vi "spurverfolgung_mit_punkten.vi"() -> ()   [LabVIEW 2014]
uses:
  <vilib>/userdefined/High Color/IMAQdx.ctl
  <vilib>/vision/driver/NI_Vision_Acquisition_Software.lvlib
  <vilib>/vision/NI_Vision_Development_Module.lvlib
panel:
  out "x":dbl
  out "y":dbl
  out "output array":dbl[][](array[numeric])
  in  "millisecond multiple":u32
  in  "größe":sgl
  out "date/time string":string
  in  "file path (dialog if empty)":path
  out "Y Resolution":i32
  out "X Resolution":i32
  in  "Template File Path (Pattern Matching 1)":path=path "C:/Users/stdekrol/Videos/patter_neu.png"
  out "Position":cluster{"x":sgl, "y":sgl}
  out "ROI":T1
  in  "Advanced Options (Pattern Matching 1)":cluster{"Item":u16, "Value":dbl}[](array[cluster])=[{"Item"=0, "Value"=10.0}, {"Item"=2, "Value"=2.0}, {"Item"=5, "Value"=300.0}, {"Item"=6, "Value"=3.0}, {"Item"=7, "Value"=5.0}, {"Item"=8, "Value"=2.0}, {"Item"=1, "Value"=1.0}, {"Item"=3, "Value"=20.0}, {"Item"=4, "Value"=0.0}] {"Item" items=["LD Sampling - Minimum Constrast"=0, "LD Sampling - Enable Subpixel Accuracy"=1, "LD Sampling - Search Strategy"=2, "LD Sampling - Subpixel Iterations"=3, "LD Sampling - Subpixel Tolerance"=4, "LD Sampling - Initial Match List Length"=5, "LD Sampling - Match List Reduction Factor"=6, "LD Sampling - Initial Step Size"=7, "LD Sampling - Intermediate Angular Accuracy"=8, "-"=9, "Pyramid - Max Pyramid Level"=100, "Pyramid - Minimum Contrast"=102, "Pyramid - Enable Subpixel Accuracy"=103, "Pyramid - Subpixel Iterations"=104, "Pyramid - Subpixel Tolerance"=105, "Pyramid - Initial Match List Length"=106, "Pyramid - Match List Reduction Factor"=107, "Pyramid - Intermediate Angular Accuracy"=108, "Pyramid - Process Border Matches"=109, "Pyramid - Min Match Separation Distance"=111, "Pyramid - Min Match Separation Angle"=112, "Pyramid - Max Match Overlap"=113, "Pyramid - Max Cache in MB"=114, "Pyramid - Clear Cache"=115]}
  in  "Parameters (Pattern Matching 1)":T2={"Number of Matches Requested"=1, "Minimum Match Score"=500.0, "Angle Ranges"=[{"Start Angle"=-180.0, "End Angle"=180.0}, {"Start Angle"=0.0, "End Angle"=360.0}]}
  in  "Algorithm (Pattern Matching 1)":i32(ring)=1 items=["All", "Low Discrepancy Sampling", "Grayscale Value Pyramid", "Gradients Pyramid"]
  out "Frame rate":dbl
  out "Matches (Pattern Matching 1)":T3(array[cluster]) {"Bounding Box"."y" format="%.2f"; "Bounding Box"."x" format="%.2f"; "Position"."y" format="%.2f"; "Position"."x" format="%.2f"; "Score" format="%.2f"; "Scale" format="%.2f"; "Angle" format="%.2f"}
  out "Number of Matches (Pattern Matching 1)":i32
  in  "stop":bool
  in  "Replace Value (1)":sgl=255.0 format="%.2f"
  in  "Threshold Limits":cluster{"Lower value":sgl, "Upper value":sgl}={"Lower value"=0.0, "Upper value"=150.0} {"Upper value" format="%.2f"; "Lower value" format="%.2f"}
  in  "Method (clustering)":i32(ring) items=["clustering", "entropy", "metric", "moments", "inter-class variance"]
  in  "Look For (Bright Objects)":u32(ring) items=["Bright Objects", "Dark Objects"]
  out "Threshold Image 2":T4(plugin-control)
  in  "Keep/Replace Value (Replace)":bool=TRUE
  out "Image 2":T4(plugin-control)
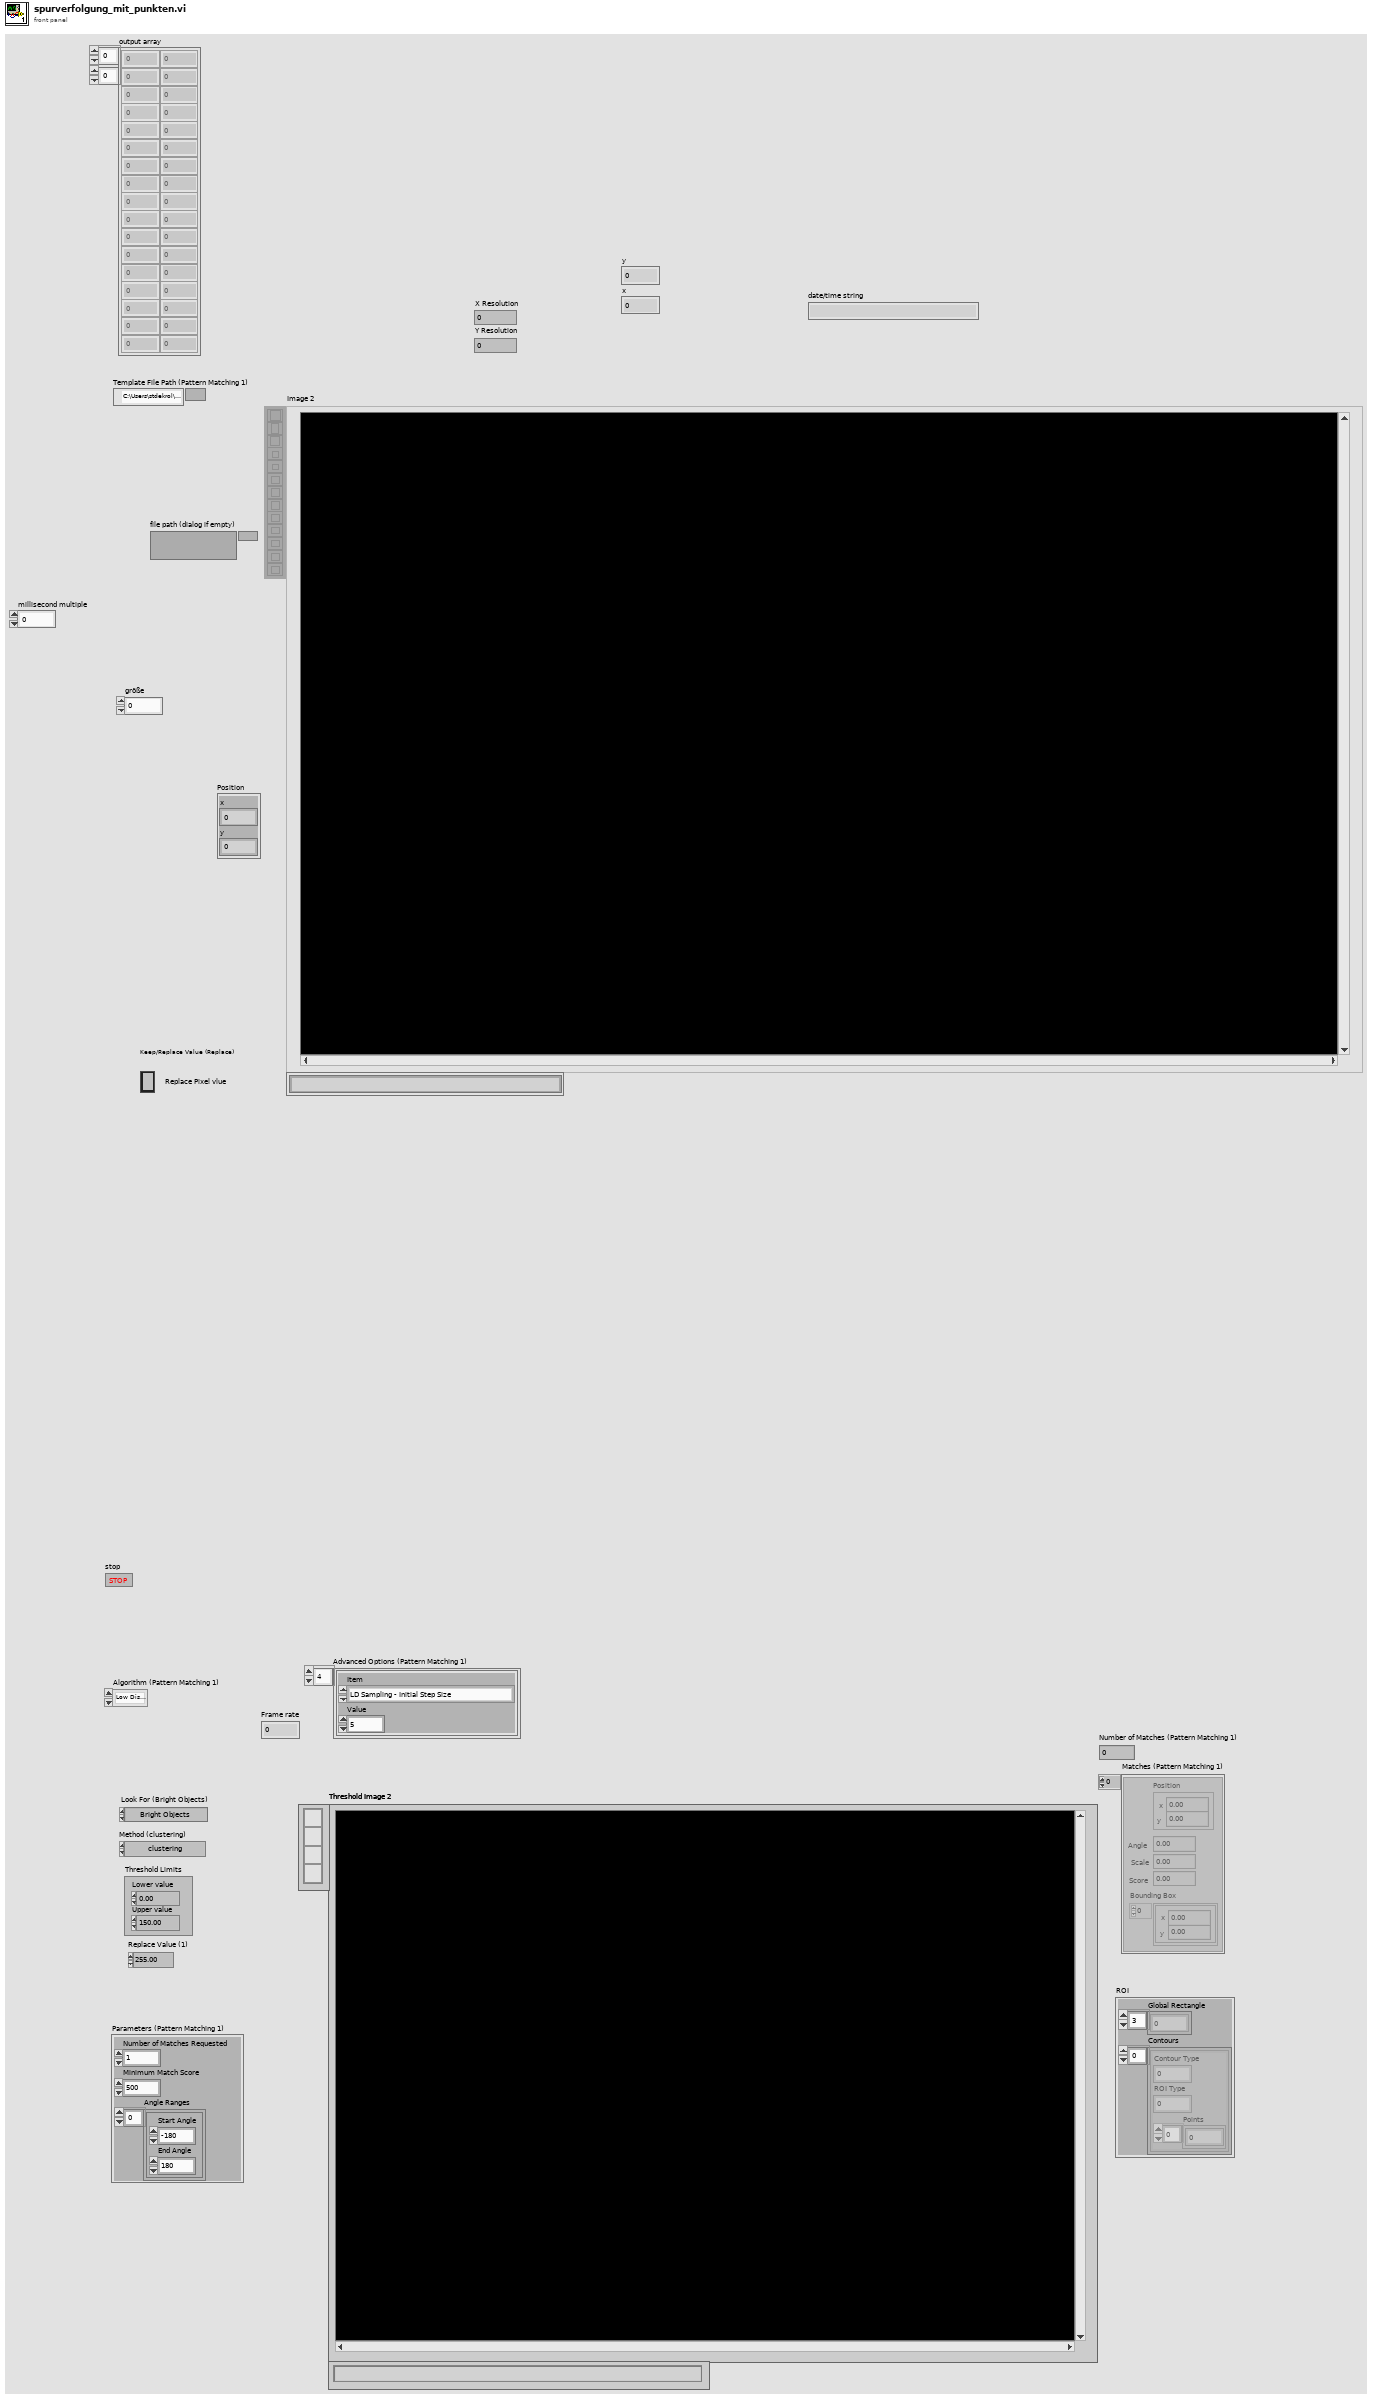
[diagram p1: front panel]
types:
  T1 = cluster{"Global Rectangle":i32[], "Contours":cluster{"Contour Type":u32, "ROI Type":u32, "Points":i32[]}[]}
  T2 = cluster{"Number of Matches Requested":i32, "Minimum Match Score":sgl, "Angle Ranges":cluster{"Start Angle":sgl, "End Angle":sgl}[]}
  T3 = cluster{"Position":cluster{"x":sgl, "y":sgl}, "Angle":sgl, "Scale":sgl, "Score":sgl, "Bounding Box":cluster{"x":sgl, "y":sgl}[]}[]
  T4 = typedef "IMAQ Image.ctl" = refnum<image>
  T5 = enum16{"open", "replace", "create", "open or create", "replace or create", "replace or create with confirmation"}
  T6 = typedef "Image Type" = u32
  T7 = typedef "IMAQdx.ctl" = refnum<k21>
  T8 = cluster{"Matches (Pattern Matching 1)[0]":cluster{"Position":cluster{"x":sgl, "y":sgl}, "Angle":sgl, "Scale":sgl, "Score":sgl, "Bounding Box":cluster{"x":sgl, "y":sgl}[]}, "Matches (Pattern Matching 1)[1]":cluster{"Position":cluster{"x":sgl, "y":sgl}, "Angle":sgl, "Scale":sgl, "Score":sgl, "Bounding Box":cluster{"x":sgl, "y":sgl}[]}, "Matches (Pattern Matching 1)[2]":cluster{"Position":cluster{"x":sgl, "y":sgl}, "Angle":sgl, "Scale":sgl, "Score":sgl, "Bounding Box":cluster{"x":sgl, "y":sgl}[]}, "Matches (Pattern Matching 1)[3]":cluster{"Position":cluster{"x":sgl, "y":sgl}, "Angle":sgl, "Scale":sgl, "Score":sgl, "Bounding Box":cluster{"x":sgl, "y":sgl}[]}, "Matches (Pattern Matching 1)[4]":cluster{"Position":cluster{"x":sgl, "y":sgl}, "Angle":sgl, "Scale":sgl, "Score":sgl, "Bounding Box":cluster{"x":sgl, "y":sgl}[]}, "Matches (Pattern Matching 1)[5]":cluster{"Position":cluster{"x":sgl, "y":sgl}, "Angle":sgl, "Scale":sgl, "Score":sgl, "Bounding Box":cluster{"x":sgl, "y":sgl}[]}, "Matches (Pattern Matching 1)[6]":cluster{"Position":cluster{"x":sgl, "y":sgl}, "Angle":sgl, "Scale":sgl, "Score":sgl, "Bounding Box":cluster{"x":sgl, "y":sgl}[]}, "Matches (Pattern Matching 1)[7]":cluster{"Position":cluster{"x":sgl, "y":sgl}, "Angle":sgl, "Scale":sgl, "Score":sgl, "Bounding Box":cluster{"x":sgl, "y":sgl}[]}, "Matches (Pattern Matching 1)[8]":cluster{"Position":cluster{"x":sgl, "y":sgl}, "Angle":sgl, "Scale":sgl, "Score":sgl, "Bounding Box":cluster{"x":sgl, "y":sgl}[]}}
  T9 = cluster{"Position":cluster{"x":sgl, "y":sgl}, "Angle":sgl, "Scale":sgl, "Score":sgl, "Bounding Box":cluster{"x":sgl, "y":sgl}[]}
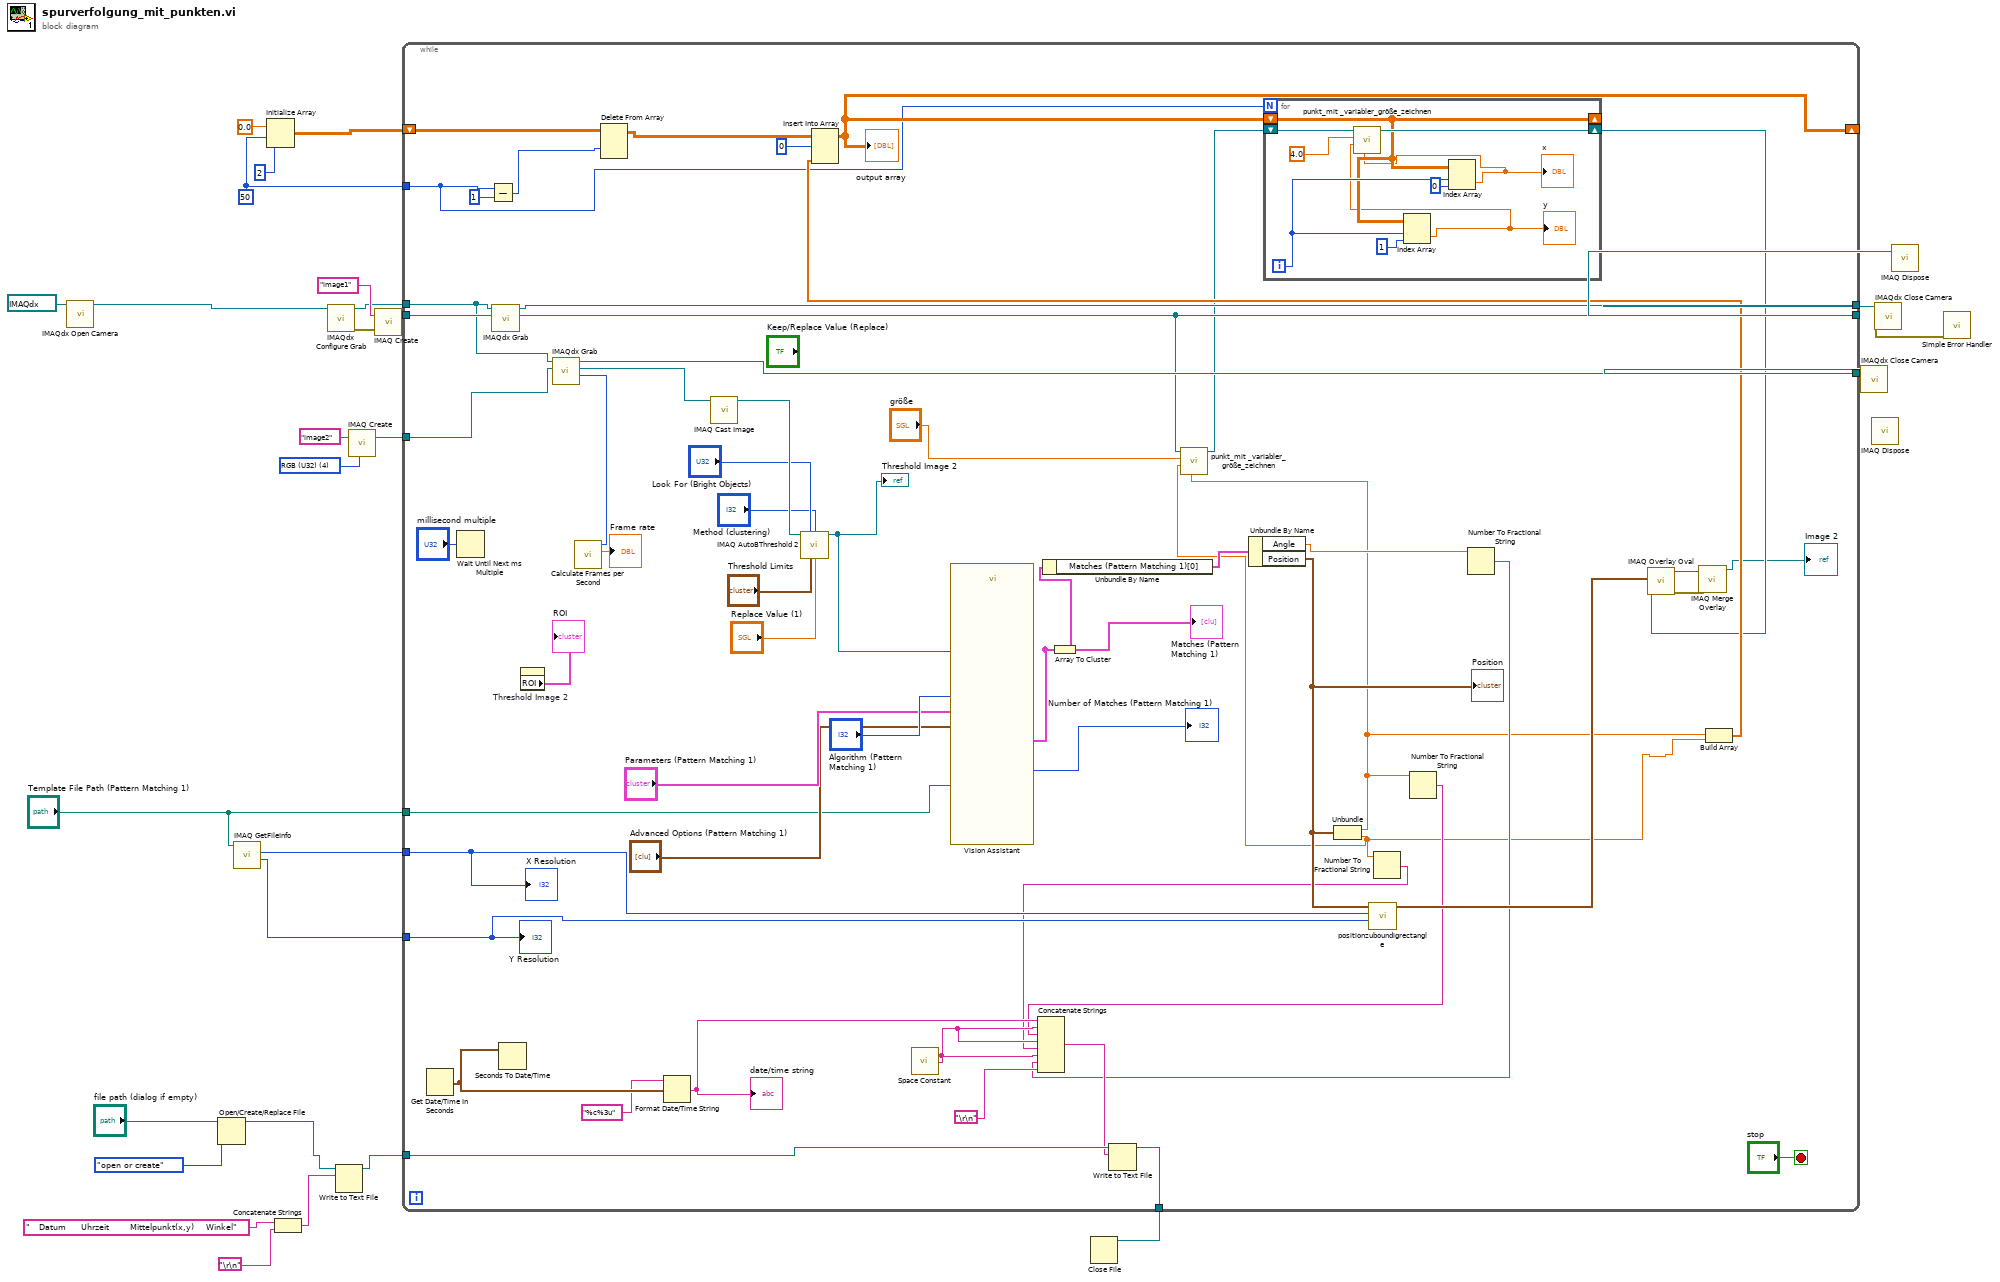
[diagram p0: block diagram]
diagram:
  w1 = 50 ("dimension size")
  w16 = T6 4 items=["Grayscale (U8)", "Grayscale (I16)", "Grayscale (SGL)", "Complex (CSG)", "RGB (U32)", "HSL (U32)", "RGB (U64)", "Grayscale (U16)"] ("Image Type")
  n1 = call <vilib>:"IMAQdx Open Camera.vi"("Session In"=T7 "cam0") -> ("Session Out"=w21:T7)  [unwired: 9 in, 1 out]
  n2 = Open/Create/Replace File(file path (use dialog)="file path (dialog if empty)", operation (0:open)=T5."open or create") -> (refnum out=w9:refnum<file>)  [unwired: 4 in, 2 out]
  n3 = call "IMAQ GetFileInfo"("File Path"="Template File Path (Pattern Matching 1)") -> ("Y Resolution"=w13:i32, "X Resolution"=w14:i32)  [unwired: 4 in, 5 out]
  n4 = Initialize Array "Initialize Array"(0.0 ("element"), w1, 2 ("dimension size")) -> (w3:dbl[][])
  n5 = Concatenate Strings("   Datum     Uhrzeit       Mittelpunkt(x,y)    Winkel" ("string"), "\r\n") -> (w5:string)
  n6 = call <vilib>:"IMAQdx Configure Grab.vi"("Session In"=w21) -> ("error out"=w27:errorcluster, "Session Out"=w25:T7)  [unwired: 9 in]
  n7 = Write to Text File(file (use dialog)=w9, text=w5) -> (refnum out=w8:refnum<file>)  [unwired: 2 in, 2 out]
  n8 = call "IMAQ Create"("Image Name"="image2", "Image Type"=w16) -> ("New Image"=w19:T4)  [unwired: 3 in, 1 out]
  n9 = call "IMAQ Create"("Image Name"="image1", "error in (no error)"=w27) -> ("New Image"=w24:T4)  [unwired: 3 in, 1 out]
  n10 = while {
    tunnel: w25 -> [w83]
    tunnel: w24 -> [w85]
    tunnel: [w86] -> w22
    tunnel: [w47] -> w17
    tunnel: w19 -> [w82]
    tunnel: [w84] -> w18
    tunnel: "Template File Path (Pattern Matching 1)" -> [w63]
    tunnel: w14 -> [w62]
    tunnel: w13 -> [w61]
    tunnel: [w58] -> w12
    tunnel: w8 -> [w57]
    shift-right: [w35] -> _
    shift-left: w3 -> [w44]
    tunnel: w1 -> [w32]
    stop <- "stop" stop-if-true
    n11 = Get Date/Time In Seconds() -> (seconds since 1Jan1904=w56:timestamp)
    n12 = Wait Until Next ms Multiple(millisecond multiple="millisecond multiple") -> ()  [unwired: 1 out]
    n13 = Subtract(x=w32, y=1) -> (x-y=w33:i32)
    n14 = call <vilib>:"IMAQdx Grab.vi"("Image In"=w85, "Session In"=w83) -> ("Image Out"=w47:T4, "Session Out"=w86:T7)  [unwired: 6 in, 2 out]
    n15 = Seconds To Date/Time(time stamp (now)=w56) -> ()  [unwired: 1 in, 1 out]
    n16 = property on="Threshold Image 2" class="ImageControl"() -> ("ROI"=→"ROI":T1)  [unwired: 2 in, 2 out]
    n17 = call <vilib>:"IMAQdx Grab.vi"("Image In"=w82, "Session In"=w83) -> ("Buffer Number Out"=w73:u32, "Image Out"=w81:T4, "Session Out"=w84:T7)  [unwired: 6 in, 1 out]
    n18 = call <vilib>:"Calculate Frames per Second.vi"("Buffer Number"=w73) -> ("Processed Frames/s"=→"Frame rate":dbl)  [unwired: 8 in, 2 out]
    n19 = Delete From Array "Delete From Array"(array=w44, index (row)=w33) -> (array with subset deleted=w43:dbl[][])  [unwired: 2 in, 1 out]
    n20 = Format Date/Time String(time format string (%c)="%c%3u", seconds (now)=w56) -> (date/time string=w54:string)  [unwired: 1 in]
    "date/time string" <- w54
    n21 = call "IMAQ Cast Image"("Image Src"=w81) -> ("Image Dst Out"=w80:T4)  [unwired: 9 in, 1 out]
    n22 = call "IMAQ AutoBThreshold 2"("Image Src"=w80, "Look For (Bright Objects)"="Look For (Bright Objects)", "Method (clustering)"="Method (clustering)", "Threshold Limits"="Threshold Limits", "Replace Value (1)"="Replace Value (1)") -> ("Image Dst Out"=w64:T4)  [unwired: 8 in, 2 out]
    "Threshold Image 2" <- w64
    n23 = call <vilib>:"Space Constant.vi"() -> ("String"=w53:string)
    n24 = call "Vision Assistant"("Image In"=w64, "Algorithm (Pattern Matching 1)"="Algorithm (Pattern Matching 1)", "Parameters (Pattern Matching 1)"="Parameters (Pattern Matching 1)", "Advanced Options (Pattern Matching 1)"="Advanced Options (Pattern Matching 1)", "Template File Path (Pattern Matching 1)"=w63) -> ("Matches (Pattern Matching 1)"=w71:T3, "Number of Matches (Pattern Matching 1)"=→"Number of Matches (Pattern Matching 1)":i32)  [unwired: 18 in, 3 out]
    "Matches (Pattern Matching 1)" <- w71
    n25 = Array To Cluster(array=w71) -> (cluster=w65:T8)
    n26 = Unbundle By Name(w65) -> ("Matches (Pattern Matching 1)[0]"=w70:T9)
    n27 = Unbundle By Name(w70) -> ("Angle"=w41:sgl, "Position"=w59:cluster{"x":sgl, "y":sgl})
    "Position" <- w59
    n28 = Unbundle(w59) -> ("x"=w38:sgl, "y"=w39:sgl)
    n29 = call "punkt_mit _variabler_größe_zeichnen.vi"("x"=w38, "y"=w39, "größe"="größe", "Refnum in"=w47) -> ("Refnum out"=w37:T4)  [unwired: 7 in]
    n30 = call "positionzuboundigrectangle.vi"("Y Resolution"=w61, "X Resolution"=w62, "Position"=w59) -> ("Cluster"=w60:cluster{dbl, dbl, dbl, dbl})  [unwired: 8 in]
    n31 = Number To Fractional String(number=w39) -> (F-format string=w49:string)  [unwired: 3 in]
    n32 = Number To Fractional String(number=w38) -> (F-format string=w50:string)  [unwired: 3 in]
    n33 = Number To Fractional String(number=w41) -> (F-format string=w48:string)  [unwired: 3 in]
    n34 = Concatenate Strings(w54, w53, w50, w53, w49, w53, w48, "\r\n") -> (w51:string)
    n35 = Write to Text File(file (use dialog)=w57, text=w51) -> (refnum out=w58:refnum<file>)  [unwired: 2 in, 2 out]
    n36 = Build Array(w38, w39) -> (w40:sgl[])
    n37 = Insert Into Array "Insert Into Array"(array=w43, index (row)=0 ("index"), new element=w40) -> (w35:dbl[][])  [unwired: 1 in]
    "output array" <- w35
    n38 = for {
      N: w32 -> [_]
      shift-right: [w94] -> w36
      shift-left: w37 -> [w95]
      shift-right: [w89] -> _
      shift-left: w35 -> [w89]
      i -> [w91]
      n39 = Index Array(array=w89, index (row)=w91, index (col)=1 ("disabled index (col)")) -> (element=w87:dbl)
      "y" <- w87
      n40 = Index Array(array=w89, index (row)=w91, index (col)=0) -> (element=w88:dbl)
      "x" <- w88
      n41 = call "punkt_mit _variabler_größe_zeichnen.vi"("x"=w88, "y"=w87, "größe"=sgl 4.0, "Refnum in"=w95) -> ("Refnum out"=w94:T4)  [unwired: 7 in]
    }
    n42 = call "IMAQ Overlay Oval"("Bounding Rectangle"=w60, "Image"=w36) -> ("error out"=w31:errorcluster, "Image Out"=w30:T4)  [unwired: 8 in]
    n43 = call "IMAQ Merge Overlay"("error in (no error)"=w31, "Image Src"=w30) -> ("Image Dst Out"=→"Image 2":T4)  [unwired: 8 in, 1 out]
    "X Resolution" <- w62
    "Y Resolution" <- w61
  }
  n44 = Close File(refnum=w12) -> ()  [unwired: 1 in, 2 out]
  n45 = call <vilib>:"IMAQdx Close Camera.vi"("Session In"=w18) -> ()  [unwired: 10 in, 1 out]
  n46 = call "IMAQ Dispose"() -> ()  [unwired: 6 in, 1 out]
  n47 = call <vilib>:"IMAQdx Close Camera.vi"("Session In"=w22) -> ("error out"=w23:errorcluster)  [unwired: 10 in]
  n48 = call "IMAQ Dispose"("Image"=w17) -> ()  [unwired: 5 in, 1 out]
  n49 = call <vilib>:"Simple Error Handler.vi"("error in (no error)"=w23) -> ()  [unwired: 4 in, 5 out]
